vi "globalSetUp.vi"(8 "error in":errorcluster, 11 "Single Core Acyclic Loopback in":refnum<class "Single Core Acyclic Loopback.lvclass">) -> (0 "error out":errorcluster, 3 "Single Core Acyclic Loopback out":refnum<class "Single Core Acyclic Loopback.lvclass">)   [LabVIEW 2020, in "Single Core Acyclic Loopback.lvclass"]
uses:
  Single Core Acyclic Loopback.lvclass
  niveristand-custom-device-testing-tools/VeriStandTestUtilities/VeriStandTestUtilities.lvlib
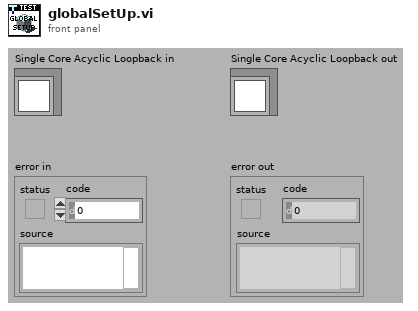
[diagram p1: front panel]
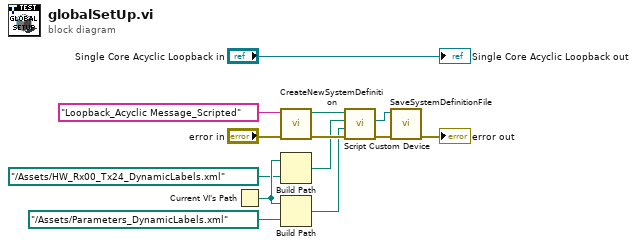
[diagram p0: block diagram]
diagram:
  n1 = Current VI's Path() -> (path=w10:path)
  n2 = call "CreateNewSystemDefinition.vi"("error in"="error in", "System Definition Name"="Loopback_Acyclic Message_Scripted" ("Channel")) -> ("error out"=w12:errorcluster, "System Definition Path"=w11:path)  [unwired: 8 in]
  n3 = Build Path(base path=w10, name or relative path=path "../Assets/HW_Rx00_Tx24_DynamicLabels.xml" ("Hardware File Path")) -> (appended path=w9:path)
  n4 = Build Path(base path=w10, name or relative path=path "../Assets/Parameters_DynamicLabels.xml" ("Hardware File Path")) -> (appended path=w8:path)
  n5 = call "Script Custom Device.vi"("error in"=w12, "Parameter File Path"=w8, "Hardware File Path"=w9, "System Definition File Path In"=w11) -> ("error out"=w3:errorcluster, "System Definition Reference"=w1:refnum<k24>)  [unwired: 4 in, 2 out]
  n6 = call "SaveSystemDefinitionFile.vi"("error in (no error)"=w3, "System Definition Reference in"=w1) -> ("error out"=→"error out":errorcluster)  [unwired: 8 in, 1 out]
  "Single Core Acyclic Loopback out" <- "Single Core Acyclic Loopback in"
